vi "Mag and Volt control.vi"() -> ()   [LabVIEW 2012]
panel:
  out "Z (uT)":dbl
  out "Y (uT)":dbl
  out "X (uT)":dbl
  in  "stop":bool
  in  "Numeric 3":dbl
  in  "Numeric 2":dbl
  in  "Numeric":dbl
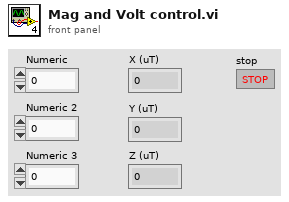
[diagram p1: front panel]
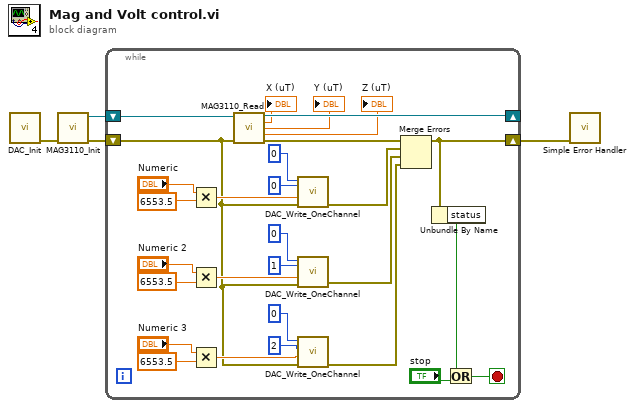
[diagram p0: block diagram]
diagram:
  n1 = call "DAC_Init.vi"() -> ("error out"=w4:errorcluster)  [unwired: 11 in]
  n2 = call "MAG3110_Init.vi"("error in (no error)"=w4) -> ("VISA resource name out"=w2:refnum<visa-resource-name>, "error out"=w3:errorcluster)  [unwired: 8 in]
  n3 = while {
    shift-right: [w32] -> _
    shift-left: w2 -> [w33]
    shift-right: [w9] -> w1
    shift-left: w3 -> [w14]
    stop <- w10 stop-if-true
    n4 = Multiply(x="Numeric", y=6553.5) -> (x*y=w26:dbl)
    n5 = Multiply(x="Numeric 2", y=6553.5) -> (x*y=w16:dbl)
    n6 = Multiply(x="Numeric 3", y=6553.5) -> (x*y=w15:dbl)
    n7 = call "MAG3110_Read.vi"("VISA resource name"=w33, "error in (no error)"=w14) -> ("VISA resource name out"=w32:refnum<visa-resource-name>, "X (uT)"=→"X (uT)":dbl, "Y (uT)"=→"Y (uT)":dbl, "Z (uT)"=→"Z (uT)":dbl, "error out"=w31:errorcluster)  [unwired: 9 in]
    n8 = call "DAC_Write_OneChannel.vi"("error in (no error)"=w14, "Value"=w26, "Channel"=u16 0, "DeviceIndex"=u64 0) -> ("error out"=w30:errorcluster)  [unwired: 6 in, 1 out]
    n9 = call "DAC_Write_OneChannel.vi"("error in (no error)"=w14, "Value"=w16, "Channel"=u16 1, "DeviceIndex"=u64 0) -> ("error out"=w13:errorcluster)  [unwired: 6 in, 1 out]
    n10 = call "DAC_Write_OneChannel.vi"("error in (no error)"=w14, "Value"=w15, "Channel"=u16 2, "DeviceIndex"=u64 0) -> ("error out"=w12:errorcluster)  [unwired: 6 in, 1 out]
    n11 = Merge Errors(w31, w30, w13, w12) -> (w9:errorcluster)
    n12 = Unbundle By Name(w9) -> ("status"=w8:bool)
    n13 = Or(x=w8, y="stop") -> (x .or. y?=w10:bool)
  }
  n14 = call <vilib>:"Simple Error Handler.vi"("error in (no error)"=w1) -> ()  [unwired: 4 in, 5 out]
